vi "Launch in separate app instances.vi"   [LabVIEW 2018, in "MQTT_Functions.lvlib"]
uses:
  MQTT_Functions.lvlib
  bb472b9f-dfe9-4ba9-8353-df3186ca7ae6.vi
types:
  T1 = cluster{"VI Path":path, "Instance Name":string}[]
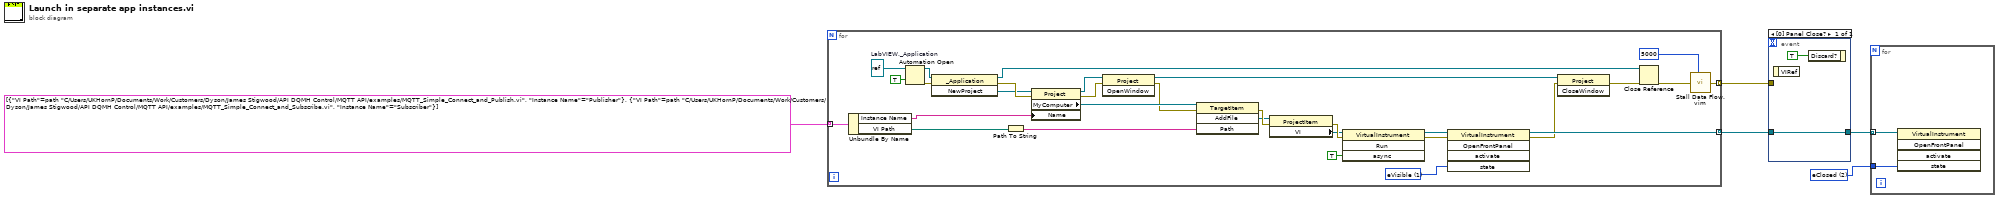
[diagram p0: block diagram]
diagram:
  w1 = 2 items=["eInvalidFPState", "eVisible", "eClosed", "eHidden", "eMinimized", "eMaximized"] ("state")
  n1 = for {
    tunnel: T1 [{"VI Path"=path "C:/Users/UKHornP/Documents/Work/Customers/Dyson/James Stigwood/API DQMH Control/MQTT API/examples/MQTT_Simple_Connect_and_Publish.vi", "Instance Name"="Publisher"}, {"VI Path"=path "C:/Users/UKHornP/Documents/Work/Customers/Dyson/James Stigwood/API DQMH Control/MQTT API/examples/MQTT_Simple_Connect_and_Subscribe.vi", "Instance Name"="Subscriber"}] -> [w34] mode=indexing
    tunnel: [w33] -> w4 mode=indexing
    tunnel: [w12] -> w3 mode=indexing
    w14 = 1 items=["eInvalidFPState", "eVisible", "eClosed", "eHidden", "eMinimized", "eMaximized"] ("state")
    w31 = refnum<k7> refnum  # LabVIEW._Application
    n2 = Unbundle By Name(w34) -> ("Instance Name"=w13:string, "VI Path"=w23:path)
    n3 = Automation Open(Automation Refnum=w31, 9:TRUE ("open new instance (false)")) -> (Automation Refnum=w30:refnum<k7>, error out=w28:errorcluster)  [unwired: 2 in]
    n4 = invoke class="_Application" method="NewProject"(reference=w30, error in=w28) -> (reference out=w26:refnum<k7>, error out=w35:errorcluster, "NewProject"=w29:refnum<k7>)  [unwired: 1 in]
    n5 = Path To String(path=w23) -> (string=w22:string)
    n6 = property class="Project"(reference=w29, error in=w35, "Name"=w13) -> (reference out=w10:refnum<k7>, error out=w11:errorcluster, "MyComputer"=w24:refnum<k7>)
    n7 = invoke class="Project" method="OpenWindow"(reference=w10, error in=w11) -> (reference out=w8:refnum<k7>, error out=w9:errorcluster)  [unwired: 1 in, 1 out]
    n8 = invoke class="TargetItem" method="AddFile"(reference=w24, error in=w9, "Path"=w22) -> (error out=w21:errorcluster, "AddFile"=w20:refnum<k7>)  [unwired: 1 in, 2 out]
    n9 = property class="ProjectItem"(reference=w20, error in=w21) -> (error out=w19:errorcluster, "VI"=w17:refnum<k7>)  [unwired: 1 out]
    n10 = invoke class="VirtualInstrument" method="Run"(reference=w17, error in=w19, "async"=TRUE) -> (reference out=w15:refnum<k7>, error out=w18:errorcluster)  [unwired: 1 in, 2 out]
    n11 = invoke class="VirtualInstrument" method="OpenFrontPanel"(reference=w15, error in=w18, "state"=w14) -> (reference out=w12:refnum<k7>, error out=w6:errorcluster)  [unwired: 2 in, 3 out]
    n12 = invoke class="Project" method="CloseWindow"(reference=w8, error in=w6) -> (error out=w7:errorcluster)  [unwired: 1 in, 2 out]
    n13 = Close Reference(reference=w26, error in (no error)=w7) -> (error out=w27:errorcluster)
    n14 = call "Stall Data Flow.vim"("value in"=w27, "milliseconds to wait"=u32 5000) -> ("value out"=w33:errorcluster)  [unwired: 1 out]
  }
  n15 = event shown="[0] Panel Close?" {
    selector: _ -> [_]
    dyn-events: _ -> [_]
    timeout: _ -> [_]
    tunnel: w4 -> [_]
    tunnel: [w36] -> w2
    tunnel: w3 -> [w36]
    event Panel Close? {
      n16 = event-data() -> ()  [unwired: 1 in, 1 out]
      n17 = event-data("Discard?"=TRUE) -> ()  [unwired: 1 in, 1 out]
    }
  }
  n18 = for {
    tunnel: w2 -> [w39] mode=indexing
    tunnel: w1 -> [w38]
    n19 = invoke class="VirtualInstrument" method="OpenFrontPanel"(reference=w39, "state"=w38) -> ()  [unwired: 3 in, 5 out]
  }
